vi "Unfill Array Len.vi"(11 "subarray":string[](array[string])) -> (3 "Len":i32)   [LabVIEW 2014]
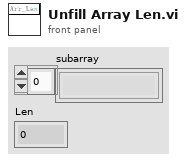
[diagram p1: front panel]
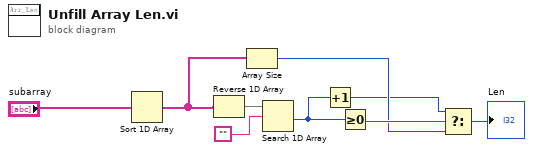
[diagram p0: block diagram]
diagram:
  n1 = Sort 1D Array(array="subarray") -> (sorted array=w8:string[])
  n2 = Reverse 1D Array(array=w8) -> (reversed array=w7:string[])
  n3 = Array Size(array=w8) -> (size(s)=w4:i32)
  n4 = Search 1D Array(1D array=w7, element="") -> (index of element=w3:i32)  [unwired: 1 in]
  n5 = Increment(x=w3) -> (x+1=w2:i32)
  n6 = Greater Or Equal To 0?(x=w3) -> (x >= 0?=w5:bool)
  n7 = Select(t=w2, s=w5, f=w4) -> (s? t:f=→"Len":i32)
